vi "rep_cap_unpack.vi"(7 "RepCap Value in":variant, 8 "error in":errorcluster, 11 "Type in":i32(ring) items=["Arbitrary", "SequentialNull", "Sequential"]) -> (0 "error out":errorcluster, 1 "RepCapCmdValues":string[](array[string]), 3 "RepCapName IDs":string[](array[string]))   [LabVIEW 2014, in "rszvl_rsidr_core.lvlib"]
uses:
  rszvl_rsidr_core.lvlib
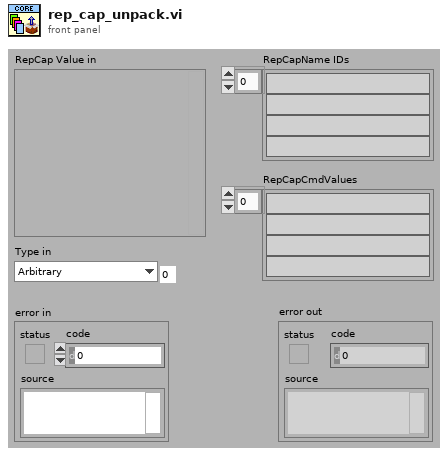
[diagram p1: front panel]
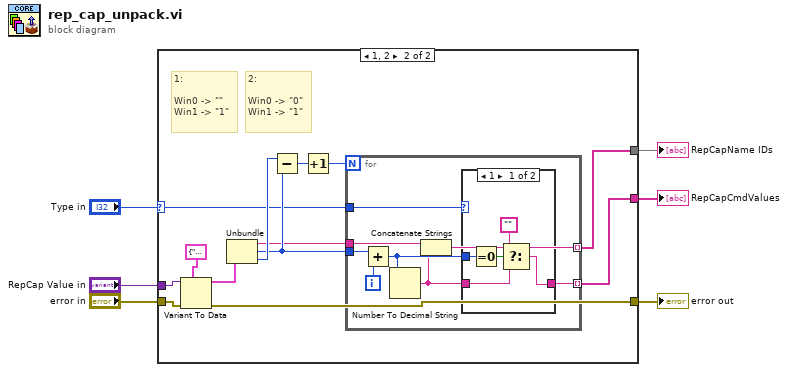
[diagram p0: block diagram]
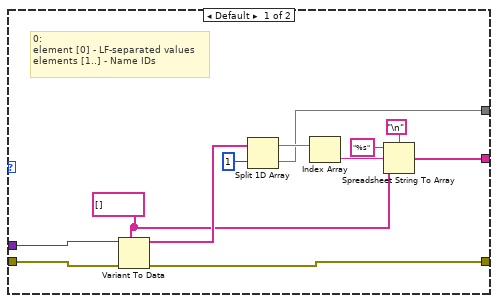
[diagram p2: hidden frame]
diagram:
  n1 = case shown="1, 2" "Type in" {
    selector: "Type in" -> [_ w23]
    tunnel: "RepCap Value in" -> [w17 w30]
    tunnel: "error in" -> [w18 w31]
    tunnel: [w16 w22] -> w5
    tunnel: [w8 w20] -> w4
    tunnel: [w7 w21] -> w3
    frame Default {
      w9 = string[] []
      # "0:\nelement [0] - LF-separated values\nelements [1..] - Name IDs"
      n2 = Variant To Data(error in=w18, type=w9, Variant=w17) -> (data=w15:string[], error out=w16:errorcluster)
      n3 = Split 1D Array(array=w15, index=1) -> (first subarray=w13:string[], second subarray=w7:string[])
      n4 = Index Array(array=w13) -> (element=w12:string)  [unwired: 1 in]
      n5 = Spreadsheet String To Array(delimiter (Tab)="\n" ("Line Feed Constant"), format string="%s", spreadsheet string=w12, array type (2D Dbl)=w9) -> (array=w8:string[])
    }
    frame 1, 2 {
      # "1:\n\nWin0 -> \"\"\nWin1 -> \"1\""
      # "2:\n\nWin0 -> \"0\"\nWin1 -> \"1\""
      n6 = Variant To Data(error in=w31, type=cluster{string, i32, i32} {"", 0, 0} ("output cluster"), Variant=w30) -> (data=w28:cluster{string, i32, i32}, error out=w22:errorcluster)
      n7 = Unbundle(w28) -> (w24:string, w25:i32, w27:i32)
      n8 = Subtract(x=w27, y=w25) -> (x-y=w26:i32)
      n9 = Increment(x=w26) -> (x+1=w19:i32)
      n10 = for {
        N: w19 -> [_]
        tunnel: w25 -> [w39]
        tunnel: w24 -> [w33]
        tunnel: w23 -> [w37]
        tunnel: [w35] -> w21 mode=indexing
        tunnel: [w34] -> w20 mode=indexing
        i -> [w38]
        n11 = Add(x=w39, y=w38) -> (x+y=w36:i32)
        n12 = Number To Decimal String(number=w36) -> (decimal integer string=w32:string)  [unwired: 1 in]
        n13 = Concatenate Strings(w33, w32) -> (w35:string)
        n14 = case shown="1" w37 {
          tunnel: w36 -> [w44 _]
          tunnel: w32 -> [w41 w45]
          tunnel: [w40 w45] -> w34
          frame 1 {
            n15 = Equal To 0?(x=w44) -> (x = 0?=w43:bool)
            n16 = Select(t="" ("Empty String Constant"), s=w43, f=w41) -> (s? t:f=w40:string)
          }
          frame 2, Default {
          }
        }
      }
    }
  }
  "error out" <- w5
  "RepCapCmdValues" <- w4
  "RepCapName IDs" <- w3
